vi "double 2 ms us ns.vi"(7 "sec":dbl format="%#_12f") -> (4 "sec":i32, 6 "ms":i32, 8 "µs":i32 min=0 max=999, 10 "ns":i32 max=999, 15 "ps":i32 max=999)   [LabVIEW 2009, in "CS POLARIS BME DG Client.lvlib"]
uses:
  CS POLARIS BME DG Client.lvlib
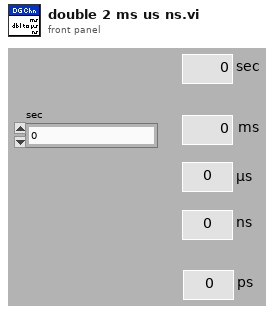
[diagram p1: front panel]
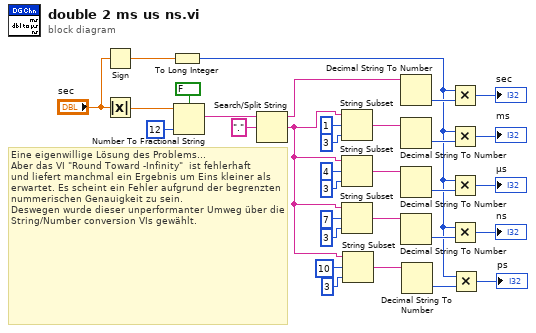
[diagram p0: block diagram]
diagram:
  # "Eine eigenwillige Lösung des Problems...\nAber das VI \"Round Toward -Infinity\"  ist fehlerhaft\nund liefert manchmal ein Ergebnis um Eins kleiner als \nerwartet. Es scheint ein Fehler aufgrund der begrenzten\nnummerischen Genauigkeit zu sein.\nDeswegen wurde dieser unperformanter Umweg über die\nString/Number conversion VIs gewählt."
  n1 = Sign(1:"sec") -> (0:w15:dbl)
  n2 = Absolute Value(x="sec") -> (abs(x)=w14:dbl)
  n3 = To Long Integer(number=w15) -> (32bit integer=w1:i32)
  n4 = Number To Fractional String(use system decimal point (T)=FALSE, number=w14, precision (6)=i16 12) -> (F-format string=w20:string)  [unwired: 1 in]
  n5 = Search/Split String(string=w20, search string/char (-)=".") -> (substring before match=w18:string, match + rest of string=w2:string)  [unwired: 1 in, 1 out]
  n6 = String Subset(string=w2, offset (0)=1, length (rest)=3 ("length (rest)")) -> (substring=w26:string)
  n7 = String Subset(string=w2, offset (0)=4, length (rest)=3 ("length (rest)")) -> (substring=w24:string)
  n8 = String Subset(string=w2, offset (0)=7 ("length (rest)"), length (rest)=3 ("offset (0)")) -> (substring=w25:string)
  n9 = String Subset(string=w2, offset (0)=10 ("length (rest)"), length (rest)=3 ("offset (0)")) -> (substring=w5:string)
  n10 = Decimal String To Number(string=w18) -> (number=w13:i32)  [unwired: 2 in, 1 out]
  n11 = Decimal String To Number(string=w26) -> (number=w12:i32)  [unwired: 2 in, 1 out]
  n12 = Decimal String To Number(string=w24) -> (number=w23:i32)  [unwired: 2 in, 1 out]
  n13 = Decimal String To Number(string=w25) -> (number=w22:i32)  [unwired: 2 in, 1 out]
  n14 = Decimal String To Number(string=w5) -> (number=w6:i32)  [unwired: 2 in, 1 out]
  n15 = Multiply(x=w1, y=w13) -> (x*y=→"sec":i32)
  n16 = Multiply(x=w1, y=w12) -> (x*y=→"ms":i32)
  n17 = Multiply(x=w1, y=w23) -> (x*y=→"µs":i32)
  n18 = Multiply(x=w1, y=w22) -> (x*y=→"ns":i32)
  n19 = Multiply(x=w1, y=w6) -> (x*y=→"ps":i32)
